vi "ReadOutSumvAD.vi"(6 "time out":u32, 10 "类型":u32(ring)=4 items=["PCI5121"=1, "PCI9810"=2, "USBCAN1"=3, "USBCAN2"=4, "PCI9820"=5, "CAN232"=6, "PCI5110"=7, "CANLite(mini)"=8, "ISA9620"=9, "ISA5420"=10, "PC104CAN"=11, "CANET"=17, "DNP9810"=13, "USBCAN-E-U"=20, "USBCAN-2E-U"=21], 12 "设备索引":u32(ring) items=["0", "1", "2", "3", "4", "5", "6", "7", "8", "9", "10", "11", "12", "13", "14", "15", ""], 16 "CAN路数":u32(ring) items=["0", "1"]) -> (20 "recv ok?":bool, 22 "AD":u16)   [LabVIEW 2013]
uses:
  AutoBurn/Settings/ControlCAN.dll
panel:
  out "VCI_CAN_OBJ_T":T1 {"ID" format="%x"}
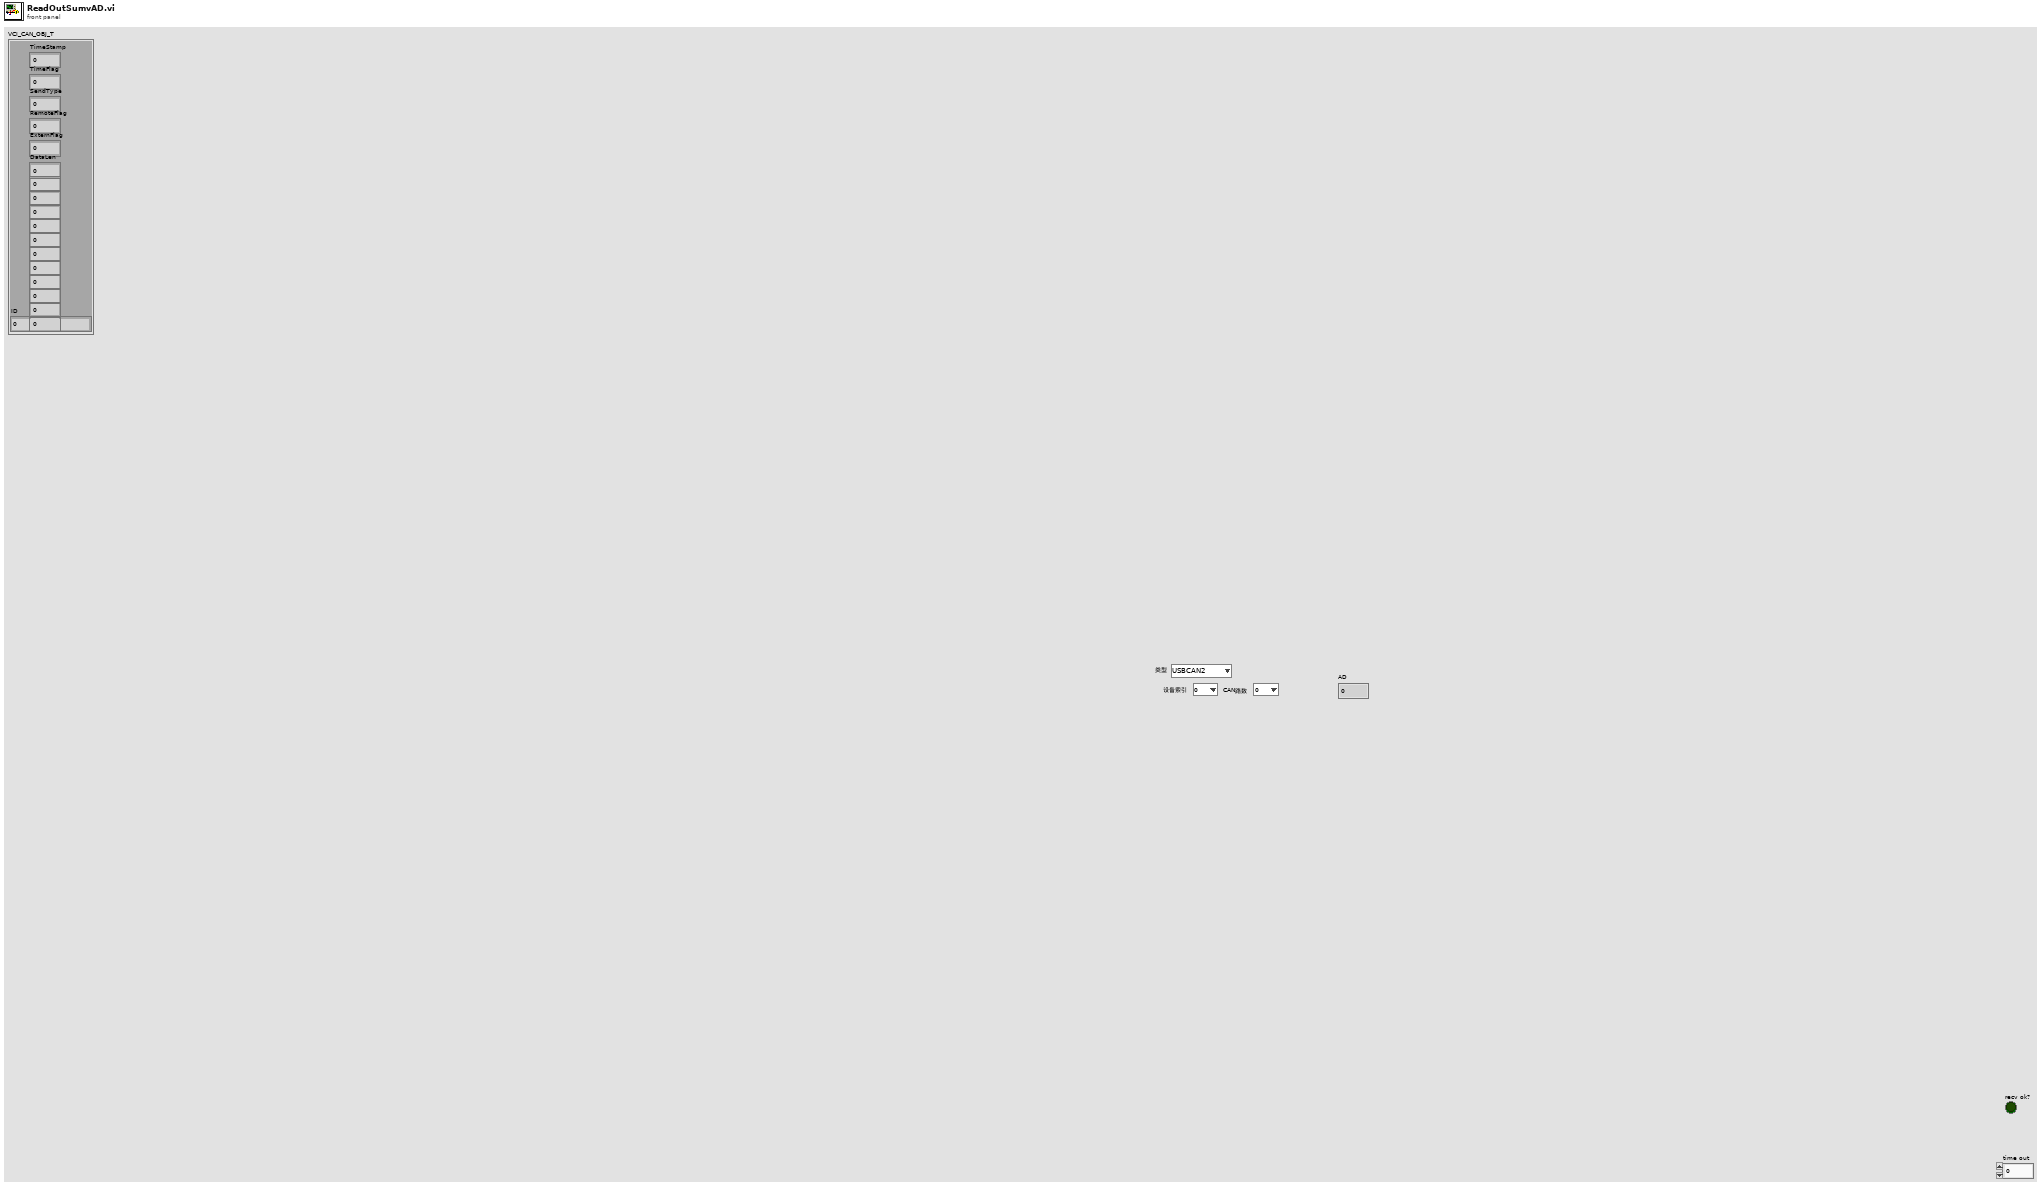
[diagram p1: front panel]
types:
  T1 = cluster{"ID":u32, "TimeStamp":u32, "TimeFlag":u8, "SendType":u8, "RemoteFlag":u8, "ExternFlag":u8, "DataLen":u8, u8, u8, u8, u8, u8, u8, u8, u8, u8, u8, u8}
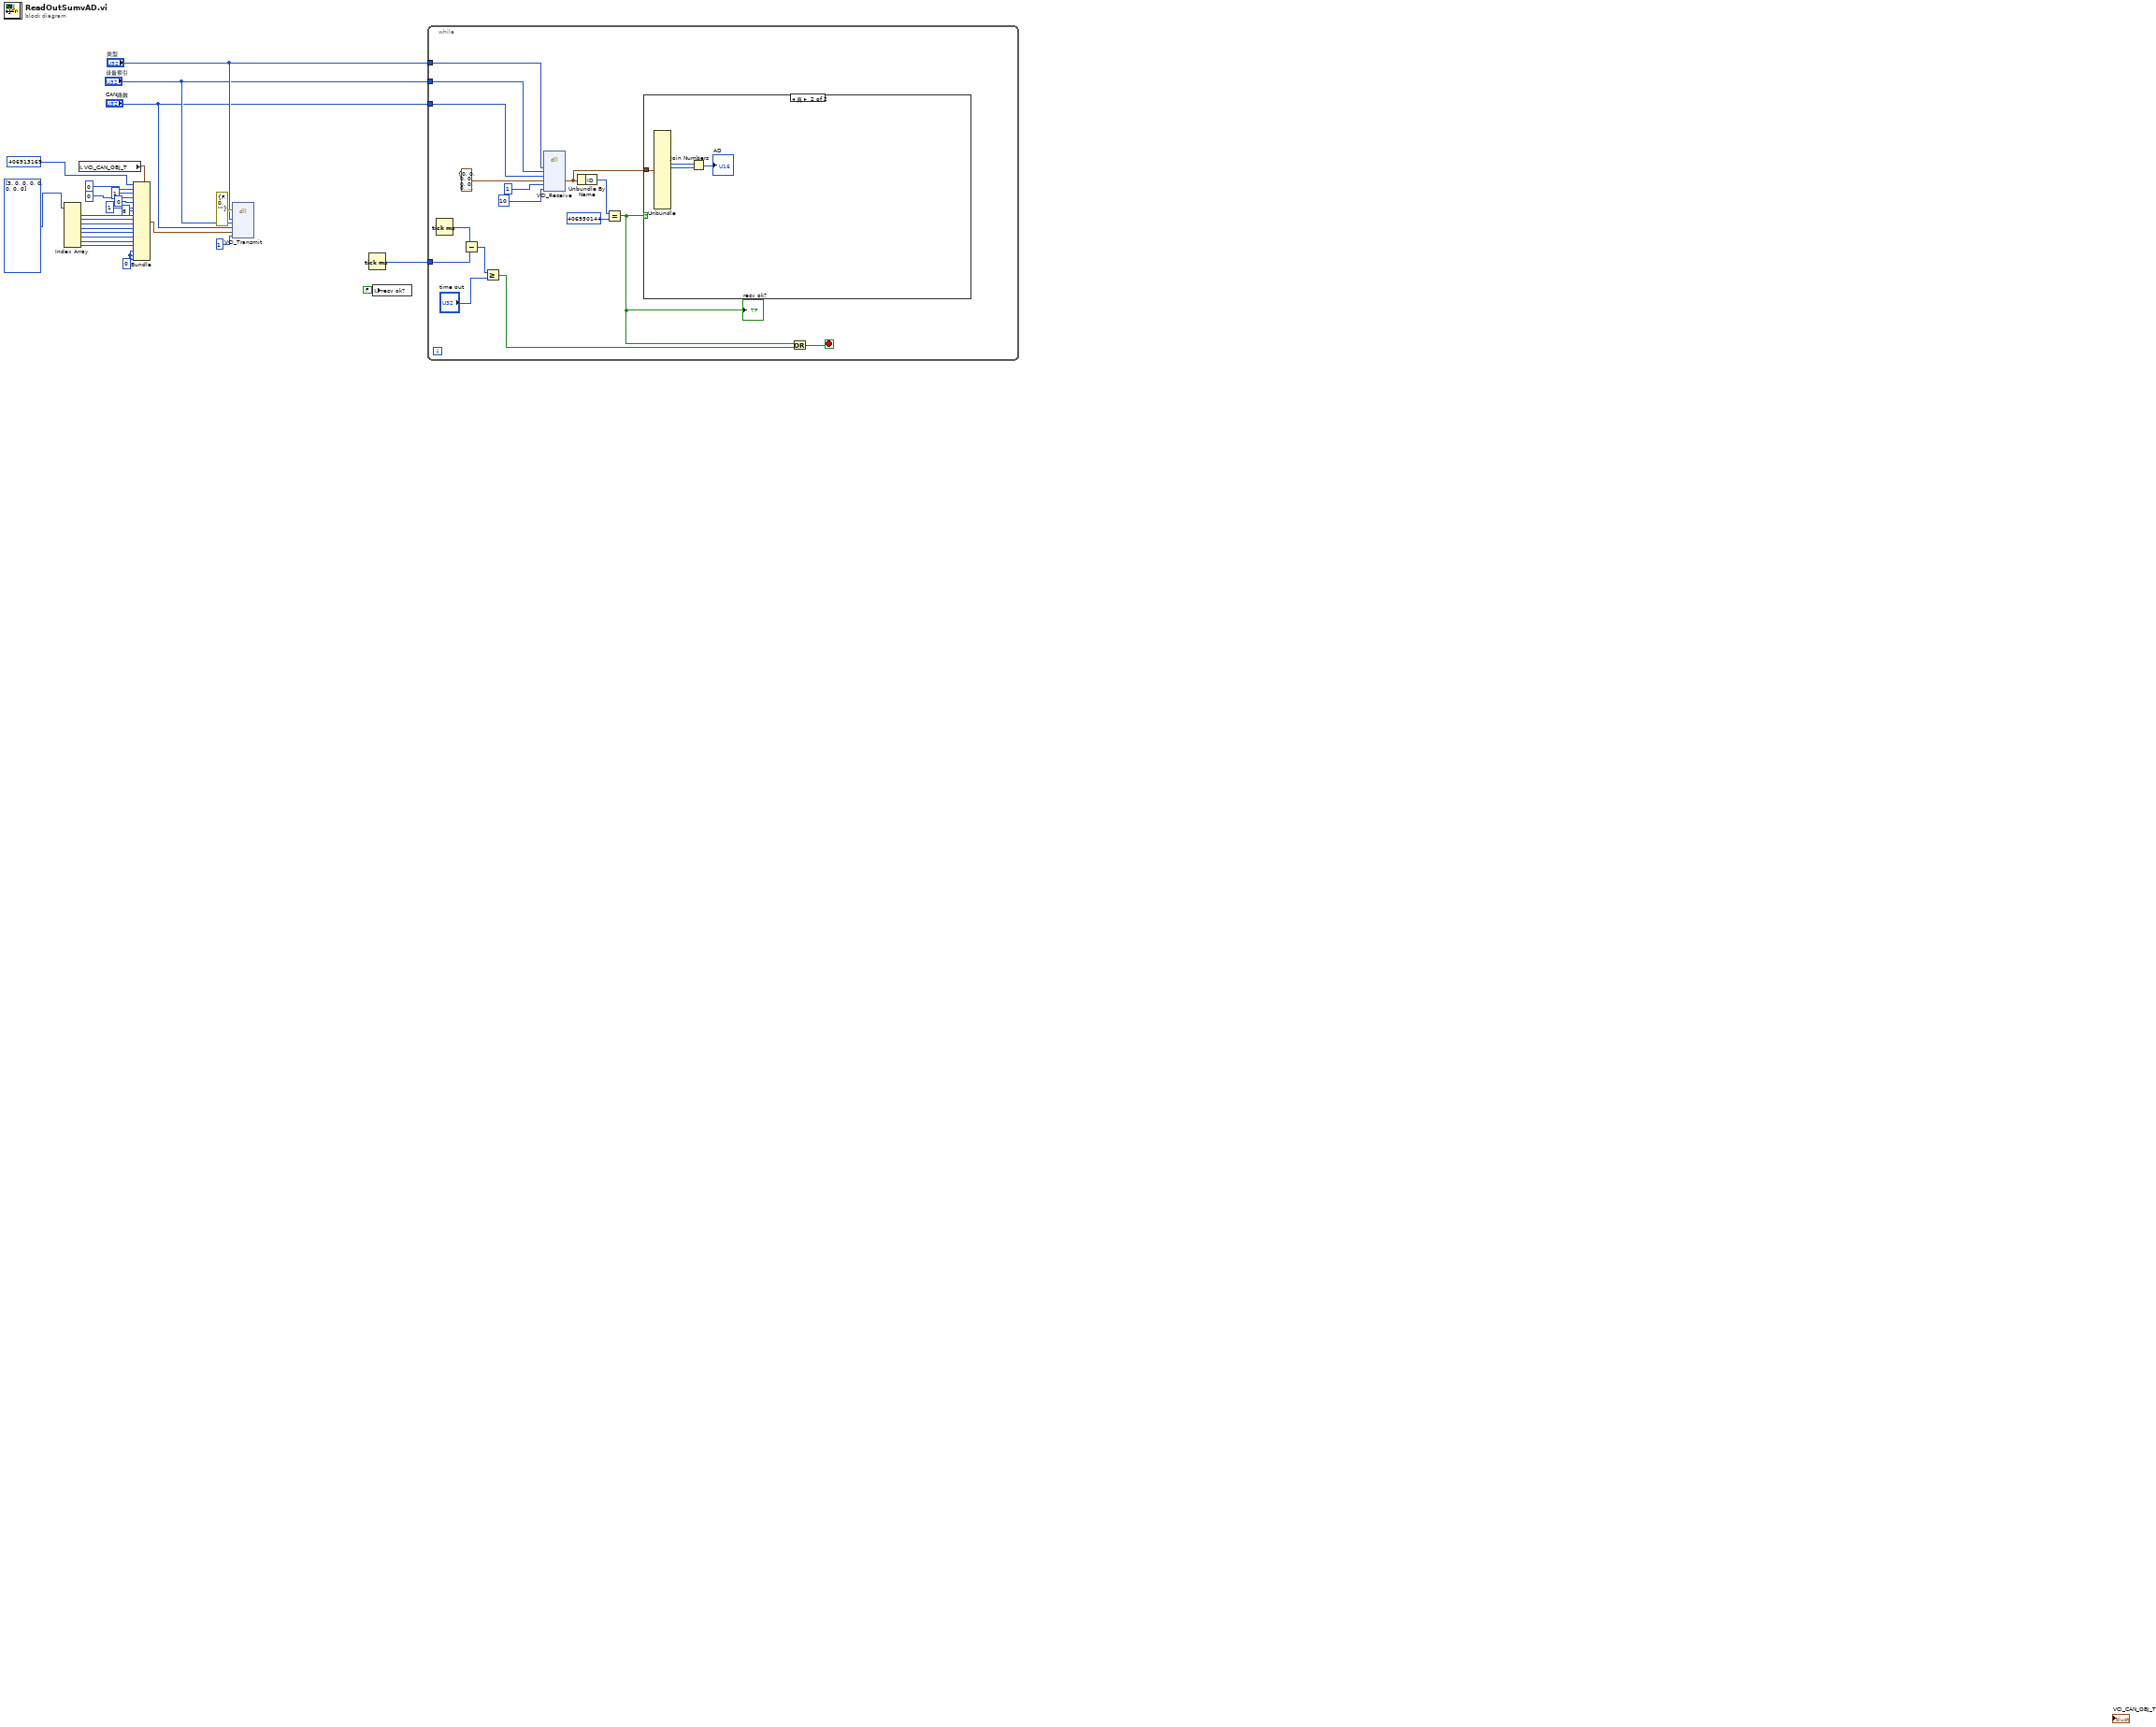
[diagram p0: block diagram]
diagram:
  w18 = u8 0 ("元素")
  n1 = Index Array(array=u8[] [3, 0, 0, 0, 0, 0, 0, 0] ("数组")) -> (element #1=w16:u8, element #2=w15:u8, element #3=w14:u8, element #4=w13:u8, element #5=w12:u8, element #6=w11:u8, element #7=w10:u8, element #8=w9:u8)  [unwired: 8 in]
  n2 = local read "VCI_CAN_OBJ_T"() -> (w22:T1)
  n3 = Bundle(cluster=w22, "ID"=u32 406913169 ("RemoteFlag"), "TimeStamp"=u8 0 ("RemoteFlag"), "TimeFlag"=u8 1, "SendType"=u8 0 ("DataLen"), "RemoteFlag"=u8 0, "ExternFlag"=u8 1, "DataLen"=u8 8, w16, w15, w14, w13, w12, w11, w10, w9, w18, w18, w18) -> (w23:T1)
  n4 = dll-call lib="F:/Bluewave New Energy/SVN_Work/AutoTest_TestStand/trunk/AutoTest_TestStand/Driver/ZlgCan/BHN01/AutoBurn/Settings/ControlCAN.dll" fn="VCI_Transmit"(error in=errorcluster {"status"=FALSE, "code"=0, "source"=""} ("错误输入（无错误）"), "DeviceType"="类型", "DeviceInd"="设备索引", "CANInd"="CAN路数", "pSend"=w23, "Len"=u32 1) -> ()  [unwired: 4 in, 6 out]
  n5 = Tick Count (ms)() -> (millisecond timer value=w26:u32)
  n6 = local write "recv ok?"(FALSE ("x = y?")) -> ()
  n7 = while {
    tunnel: w26 -> [w38]
    tunnel: "类型" -> [w29]
    tunnel: "设备索引" -> [w28]
    tunnel: "CAN路数" -> [w27]
    stop <- w32 stop-if-true
    n8 = Tick Count (ms)() -> (millisecond timer value=w39:u32)
    n9 = Subtract(x=w39, y=w38) -> (x-y=w37:u32)
    n10 = Greater Or Equal?(x=w37, y="time out") -> (x >= y?=w33:bool)
    n11 = dll-call lib="F:/Bluewave New Energy/SVN_Work/AutoTest_TestStand/trunk/AutoTest_TestStand/Driver/ZlgCan/BHN01/AutoBurn/Settings/ControlCAN.dll" fn="VCI_Receive"("DeviceType"=w29, "DeviceInd"=w28, "CANInd"=w27, "pReceive"=T1 {"ID"=0, "TimeStamp"=0, "TimeFlag"=0, "SendType"=0, "RemoteFlag"=0, "ExternFlag"=0, "DataLen"=0, 0, 0, 0, 0, 0, 0, 0, 0, 0, 0, 0}, "Len"=u32 1, "WaitTime"=10) -> ("pReceive"=w31:T1)  [unwired: 8 in, 3 out]
    n12 = Unbundle By Name(w31) -> ("ID"=w35:u32)
    n13 = Equal?(x=w35, y=u32 406950144) -> (x = y?=w34:bool)
    "recv ok?" <- w34
    n14 = case shown="真" w34 {
      tunnel: w31 -> [_ w46]
      frame False {
      }
      frame True {
        n15 = Unbundle(w46) -> (w45:u8, w44:u8)  [unwired: 16 out]
        n16 = Join Numbers(hi=w45, lo=w44) -> ((hi.lo)=→"AD":u16)
      }
    }
    n17 = Or(x=w34, y=w33) -> (x .or. y?=w32:bool)
  }
